vi "launcher.vi"() -> ()   [LabVIEW 2020]
panel:
  in  "Boolean":bool
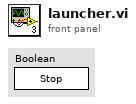
[diagram p1: front panel]
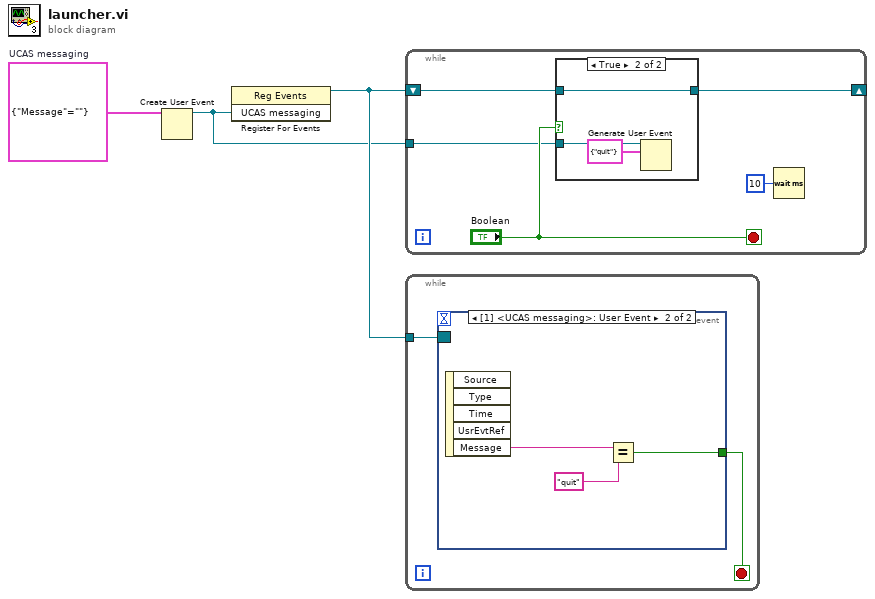
[diagram p0: block diagram]
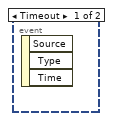
[diagram p2: hidden frame]
diagram:
  w3 = cluster{"Message":string} {"Message"=""}  # UCAS messaging
  n1 = Create User Event(user event datatype=w3) -> (user event=w1:refnum<user-event>)  [unwired: 1 in, 1 out]
  n2 = register-events(w1) -> (reference out=w2:refnum<event-registration>)  [unwired: 2 in, 1 out]
  n3 = while {
    shift-right: [w5] -> _
    shift-left: w2 -> [w6]
    tunnel: w1 -> [w4]
    stop <- "Boolean" stop-if-true
    n4 = case shown="True" "Boolean" {
      tunnel: w6 -> [w9 w12]
      tunnel: [w9 w12] -> w5
      tunnel: w4 -> [_ w11]
      frame False {
      }
      frame True {
        n5 = Generate User Event(user event=w11, event data cluster=cluster{"Message":string} {"Message"="quit"} ("event data")) -> ()  [unwired: 2 in, 2 out]
      }
    }
    n6 = Wait (ms)(milliseconds to wait=u32 10) -> ()  [unwired: 1 out]
  }
  n7 = while {
    tunnel: w2 -> [w14]
    stop <- w13 stop-if-true
    n8 = event shown="[1] <UCAS messaging>: User Event" {
      selector: w14 -> [_ _]
      dyn-events: _ -> [_ _]
      timeout: _ -> [_ _]
      tunnel: [_ w15] -> w13
      event Timeout {
        n9 = event-data() -> ()  [unwired: 1 in, 3 out]
      }
      event User Event {
        n10 = event-data() -> ("Message"=w17:string)  [unwired: 1 in, 4 out]
        n11 = Equal?(x=w17, y="quit") -> (x = y?=w15:bool)
      }
    }
  }
